vi "NF90 Home.vi"(5 "Index offset from switch":sgl min=-1048575 max=1048575 step=1 format="%.2f", 7 "Error In":errorcluster, 9 "move":T1={"axis"=enum."X", "Increment"=0.0, "Speed"=1.0, "Acceleration"=1} {"Speed" min=0 format="%.3f"; "Acceleration" min=1 max=50 step=1; "Increment" format="%.3f"}, 10 "port number in":refnum<visa-resource-name>) -> (0 "Error Out":errorcluster, 1 "killed":bool, 2 "position":dbl format="%.2f", 3 "port number out":refnum<visa-resource-name>)   [LabVIEW 2012]
uses:
  NF90 move.ctl
  Axis.ctl
  NF90 commands.ctl
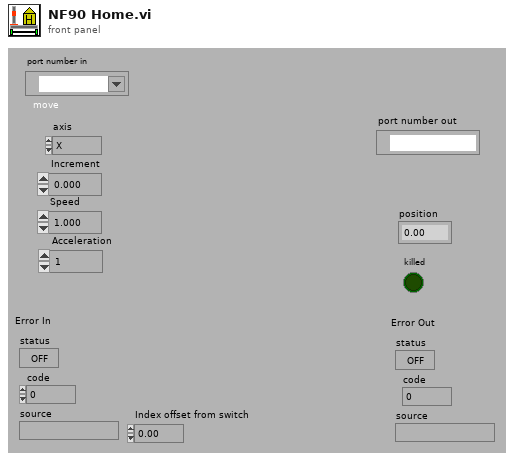
[diagram p1: front panel]
types:
  T1 = typedef "NF90 move.ctl" = cluster{"axis":T2, "Increment":sgl, "Speed":sgl, "Acceleration":u8}
  T2 = typedef "Axis.ctl" = enum16{"X", "Y", "Z"}
  T3 = typedef "NF90 commands.ctl" = enum16{"Index", "Speed", "Acceleration", "Backlash", "Quit", "Run", "Null indexes", "Verify status", "Clear program", "Computer Control", "Go", "Put Controller on Hold", "Position"}
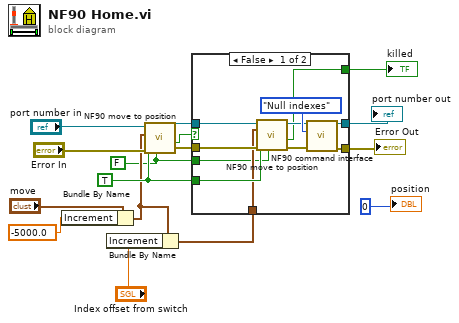
[diagram p0: block diagram]
diagram:
  w4 = FALSE ("program (Run=False)")
  w11 = TRUE ("move type")
  n1 = Bundle By Name(cluster="move", "Increment"=sgl -5000.0) -> (w6:T1)
  n2 = Bundle By Name(cluster=w6, "Increment"="Index offset from switch") -> (w9:T1)
  n3 = call "NF90 move to position.vi"("program (Run=False)"=w4, "Error In"="Error In", "move type (abs = False)"=w11, "move"=w6, "port number in"="port number in") -> ("Error Out"=w16:errorcluster, "killed"=w2:bool, "port number out"=w15:refnum<visa-resource-name>)  [unwired: 2 in, 1 out]
  n4 = case shown="False" w2 {
    selector: w2 -> [_ w28]
    tunnel: w16 -> [w27 w30]
    tunnel: w15 -> [w23 w29]
    tunnel: [w22 w30] -> w12
    tunnel: w11 -> [w21 _]
    tunnel: [w20 w29] -> w10
    tunnel: w9 -> [w19 _]
    tunnel: w4 -> [w18 _]
    tunnel: [w17 w28] -> w1
    frame False {
      n5 = call "NF90 move to position.vi"("program (Run=False)"=w18, "Error In"=w27, "move type (abs = False)"=w21, "move"=w19, "port number in"=w23) -> ("Error Out"=w26:errorcluster, "killed"=w17:bool, "port number out"=w24:refnum<visa-resource-name>)  [unwired: 2 in, 1 out]
      n6 = call "NF90 command interface.vi"("port number in"=w24, "commands"=NF90_commands."Null indexes", "Error In"=w26) -> ("port number out"=w20:refnum<visa-resource-name>, "Error Out"=w22:errorcluster)  [unwired: 8 in, 3 out]
    }
    frame True {
    }
  }
  "port number out" <- w10
  "Error Out" <- w12
  "killed" <- w1
  "position" <- 0
